vi "Select Class.vi"(7 "Class Type":T1, 8 "error in":errorcluster, 10 "Class Name":string="NI DMM4072.lvclass", 11 "Base Path":path=path "C:/GitHub/OOP_OPC UA/Sequence/CodeModules/HAL/Concrete") -> (0 "error out":errorcluster, 3 "specific class reference":refnum<class>)   [LabVIEW 2021]
uses:
  Controls/Select Class Type.ctl
  HAL/Harware Abstraction/Hardware/Instrument.lvclass
  OPC UA/OPC UA.lvclass
  HAL/Harware Abstraction/MultiIO/DMM.lvclass
  HAL/Harware Abstraction/ACIR/ACIR.lvclass
  HAL/Harware Abstraction/HiPOT/HiPOT.lvclass
  HAL/Harware Abstraction/AnalogIO/Power Supply.lvclass
  HAL/Harware Abstraction/DIO/DIO.lvclass
  HAL/Harware Abstraction/Switch/Switch.lvclass
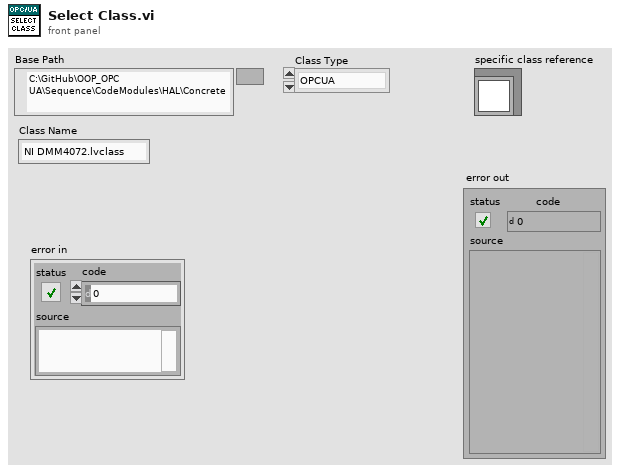
[diagram p1: front panel]
types:
  T1 = typedef "Select Class Type.ctl" = enum16{"OPCUA", "PS", "DMM", "Switch", "DIO", "HiPOT", "ACIR"}
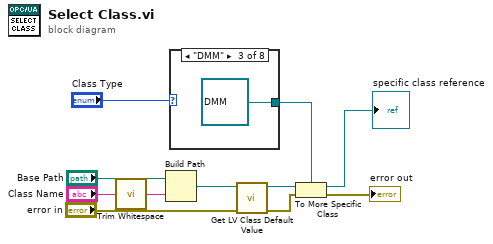
[diagram p0: block diagram]
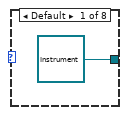
[diagram p2: hidden frame]
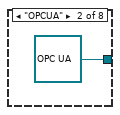
[diagram p3: hidden frame]
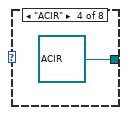
[diagram p4: hidden frame]
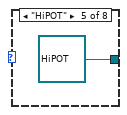
[diagram p5: hidden frame]
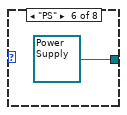
[diagram p6: hidden frame]
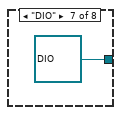
[diagram p7: hidden frame]
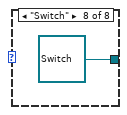
[diagram p8: hidden frame]
diagram:
  n1 = call <vilib>:"Trim Whitespace.vi"("string"="Class Name") -> ("trimmed string"=w3:string)  [unwired: 1 in]
  n2 = Build Path(base path="Base Path", name or relative path=w3) -> (appended path=w6:path)
  n3 = case shown="\"DMM\"" "Class Type" {
    tunnel: [refnum<class "Instrument.lvclass"> refnum ("HAL.lvlib:Instrument.lvclass") refnum<class "OPC UA.lvclass"> refnum ("OPC UA.lvclass") refnum<class "DMM.lvclass"> refnum ("HAL.lvlib:MultiFunction IO.lvclass") refnum<class "ACIR.lvclass"> refnum ("HAL.lvlib:ACIR.lvclass") refnum<class "HiPOT.lvclass"> refnum ("HAL.lvlib:HiPOT.lvclass") refnum<class "Power Supply.lvclass"> refnum ("HAL.lvlib:AIO.lvclass") refnum<class "DIO.lvclass"> refnum ("HAL.lvlib:DIO.lvclass") refnum<class "Switch.lvclass"> refnum ("HAL.lvlib:Switch.lvclass")] -> w10
    frame Default {
    }
    frame "OPCUA" {
    }
    frame "DMM" {
    }
    frame "ACIR" {
    }
    frame "HiPOT" {
    }
    frame "PS" {
    }
    frame "DIO" {
    }
    frame "Switch" {
    }
  }
  n4 = call <vilib>:"Get LV Class Default Value.vi"("error in (no error)"="error in", "class path"=w6) -> ("error out"=w9:errorcluster, "object"=w8:refnum<class>)  [unwired: 8 in]
  n5 = To More Specific Class(target class=w10, reference=w8, error in=w9) -> (specific class reference=→"specific class reference":refnum<class>, error out=→"error out":errorcluster)
